vi "SS2 Live_Update Image ROI Information.vi"(8 "Error In":errorcluster, 9 "Element Changed":string, 11 "Image Information Refnum":refnum<vi>) -> (0 "Error Out":errorcluster, 1 "Image Information":T1)   [LabVIEW 2019]
uses:
  SS2 Live_Image ROI Information.ctl
  SS2 Live_Settings List.ctl
  SS2 Live_Internal Data List.ctl
  Image/Image ROI Type.ctl
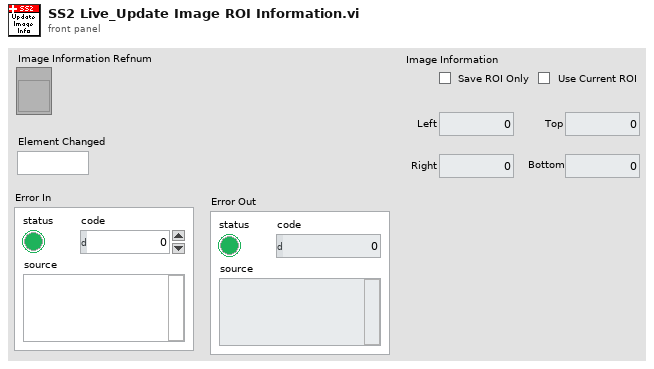
[diagram p1: front panel]
types:
  T1 = typedef "SS2 Live_Image ROI Information.ctl" = cluster{"Save ROI Only":bool, "Left":u16, "Top":u16, "Right":u16, "Bottom":u16, "Use Current ROI":bool}
  T2 = typedef "SS2 Live_Settings List.ctl" = enum16{"FPGA:Bitfile Path", "FPGA:Bitfile Version", "Acquisition Parameters:SS2 DAQ Parameters", "Acquisition Parameters:Gate Configuration Array", "Acquisition Parameters:Buffer Size (# Gates)", "File Information:File Information", "File Information:# Datasets in Series", "Image Parameters:Image ROI Information", "Image Parameters:Image Binning Options", "UI Parameters:Histogram Bins Number"}
  T3 = typedef "SS2 Live_Image Information.ctl" = cluster{"Save ROI Only":bool, "Left":u16, "Top":u16, "Right":u16, "Bottom":u16, "Use Current ROI":bool}
  T4 = typedef "Image ROI Type.ctl" = enum16{"No Selection", "Point", "Line", "Rectangle", "Oval", "Polygon", "Freehand Region", "Annulus", "Unused2", "Unused3", "Broken Line", "Freehand Line", "Rotated Rectangle"}
  T5 = typedef "SS2 Live_Internal Data List.ctl" = enum16{"Number of pending file saving tasks", "File Saving Tasks Information", "Current Image ROI Information"}
  T6 = typedef "ROI Descriptor" = cluster{"Global Rectangle":i32[], "Contours":cluster{"ID":enum32{"External", "Internal"}, "Type":u32, "Coordinates":i32[]}[]}
  T7 = cluster{"ID":enum32{"External", "Internal"}, "Type":u32, "Coordinates":i32[]}[]
  T8 = cluster{"ID":enum32{"External", "Internal"}, "Type":u32, "Coordinates":i32[]}
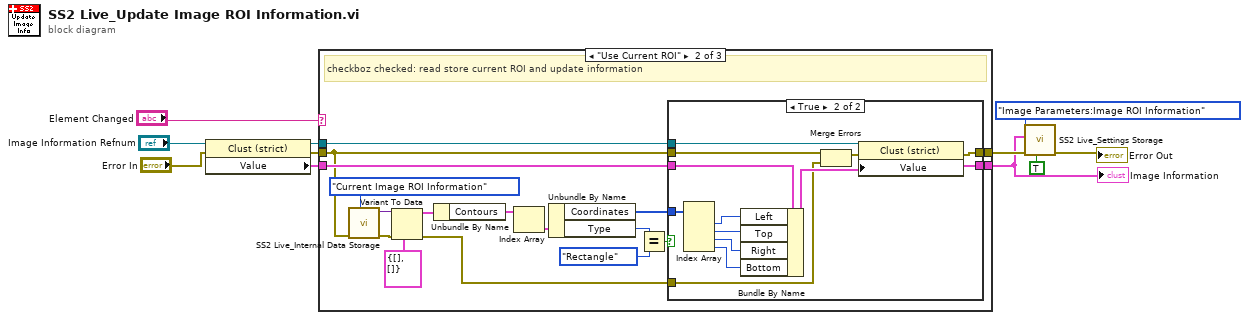
[diagram p0: block diagram]
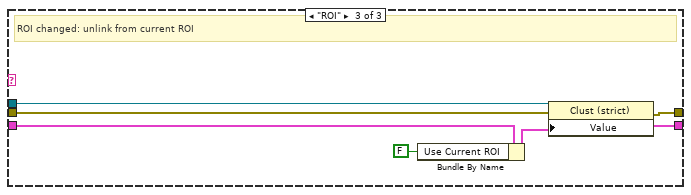
[diagram p4: hidden frame]
diagram:
  n1 = property class="Clust (strict)"(reference="Image Information Refnum", error in="Error In") -> (reference out=w10:refnum<vi>, error out=w9:errorcluster, "Value"=w2:T3)
  n2 = case shown="\"Use Current ROI\"" "Element Changed" {
    tunnel: w10 -> [_ w21 w50]
    tunnel: w9 -> [w12 w14 w49]
    tunnel: [w12 w19 w48] -> w7
    tunnel: [w13 w18 w47] -> w4
    tunnel: w2 -> [w13 w17 w46]
    frame "Only Save ROI", Default {
      # "update chackbox"
    }
    frame "Use Current ROI" {
      # "checkboz checked: read store current ROI and update information"
      n3 = call "SS2 Live_Internal Data Storage.vi"("SS2 Live Data"=SS2_Live_Internal_Data_List."Current Image ROI Information", "Error In"=w14) -> ("Error Out"=w29:errorcluster, "Variant"=w28:variant)  [unwired: 7 in, 1 out]
      n4 = Variant To Data(error in=w29, type=T6 {"Global Rectangle"=[], "Contours"=[]} ("ROI Descriptor"), Variant=w28) -> (data=w26:T6, error out=w20:errorcluster)
      n5 = Unbundle By Name(w26) -> ("Contours"=w25:T7)
      n6 = Index Array(array=w25) -> (element=w22:T8)  [unwired: 1 in]
      n7 = Unbundle By Name(w22) -> ("Coordinates"=w16:i32[], "Type"=w24:u32)
      n8 = Equal?(x=w24, y=Image_ROI_Type."Rectangle" ("ROI Type")) -> (x = y?=w15:bool)
      n9 = case shown="True" w15 {
        tunnel: w21 -> [_ w44]
        tunnel: w16 -> [_ w43]
        tunnel: w14 -> [w32 w38]
        tunnel: [w32 w37] -> w19
        tunnel: w17 -> [w31 w36]
        tunnel: [w31 w35] -> w18
        tunnel: w20 -> [_ w33]
        frame False {
        }
        frame True {
          n10 = Index Array(array=w43) -> (element #1=w42:i32, element #2=w41:i32, element #3=w40:i32, element #4=w39:i32)  [unwired: 4 in]
          n11 = Bundle By Name(cluster=w36, "Left"=w42, "Top"=w41, "Right"=w40, "Bottom"=w39) -> (w35:T3)
          n12 = Merge Errors(w38, w33) -> (w34:errorcluster)
          n13 = property class="Clust (strict)"(reference=w44, error in=w34, "Value"=w35) -> (error out=w37:errorcluster)  [unwired: 1 out]
        }
      }
    }
    frame "ROI" {
      # "ROI changed: unlink from current ROI"
      n14 = Bundle By Name(cluster=w46, "Use Current ROI"=FALSE) -> (w47:T3)
      n15 = property class="Clust (strict)"(reference=w50, error in=w49, "Value"=w47) -> (error out=w48:errorcluster)  [unwired: 1 out]
    }
  }
  "Image Information" <- w4
  n16 = call "SS2 Live_Settings Storage.vi"("Set/Get(F)"=TRUE, "Error In"=w7, "Variant Data in"=w4, "Settings List"=SS2_Live_Settings_List."Image Parameters:Image ROI Information") -> ("Error Out"=→"Error Out":errorcluster)  [unwired: 6 in, 1 out]
